vi "EyeFileExtraction.vi"() -> ()   [LabVIEW 2022 SP3]
uses:
  ViewData/-ReadEye/Header.ctl
  <vilib>/Utility/file.llb/Read Delimited Spreadsheet (string).vi
  <vilib>/Utility/file.llb/Read Delimited Spreadsheet (DBL).vi
  <userlib>/_OpenG.lib/array/array.llb/Sort 2D Array (DBL)__ogtk.vi
panel:
  in  "Save Folder Name":string="EyeFiles"
  in  "Only Real of Sum?":bool
  in  "Cut off":i32=50000
  in  "save folder path":path
  in  "Folder Override?":bool
  in  "Save All?":bool
  out "time diff":sgl[](graph)
  out "time stamp":sgl[](graph)
  in  "Split files?":bool
  out "Current File":string
  in  "IQ source":enum32{"GPU", "Verasonics", "None"}(radio)
  out "Current File Ct":i32
  in  "Enum":T1(ring)
  out "Header Size":i32[](array[numeric])
  out "Header clolumn names":string[](array[string])
  in  "Header as cluster":T2
  out "Header Values sorted":dbl[][](array[numeric])
  in  "Use Selected Files":bool
  in  "Listbox":i32[](listbox)
  in  "directory path of data and header file":path
  in  "search pattern":string="*_HeaderInfoRcv.txt"
  # "Naming must match up\nDo not change order in Matlab save !!!!!!!!!!!!!!!!!!!!!!!!!!!!!!"
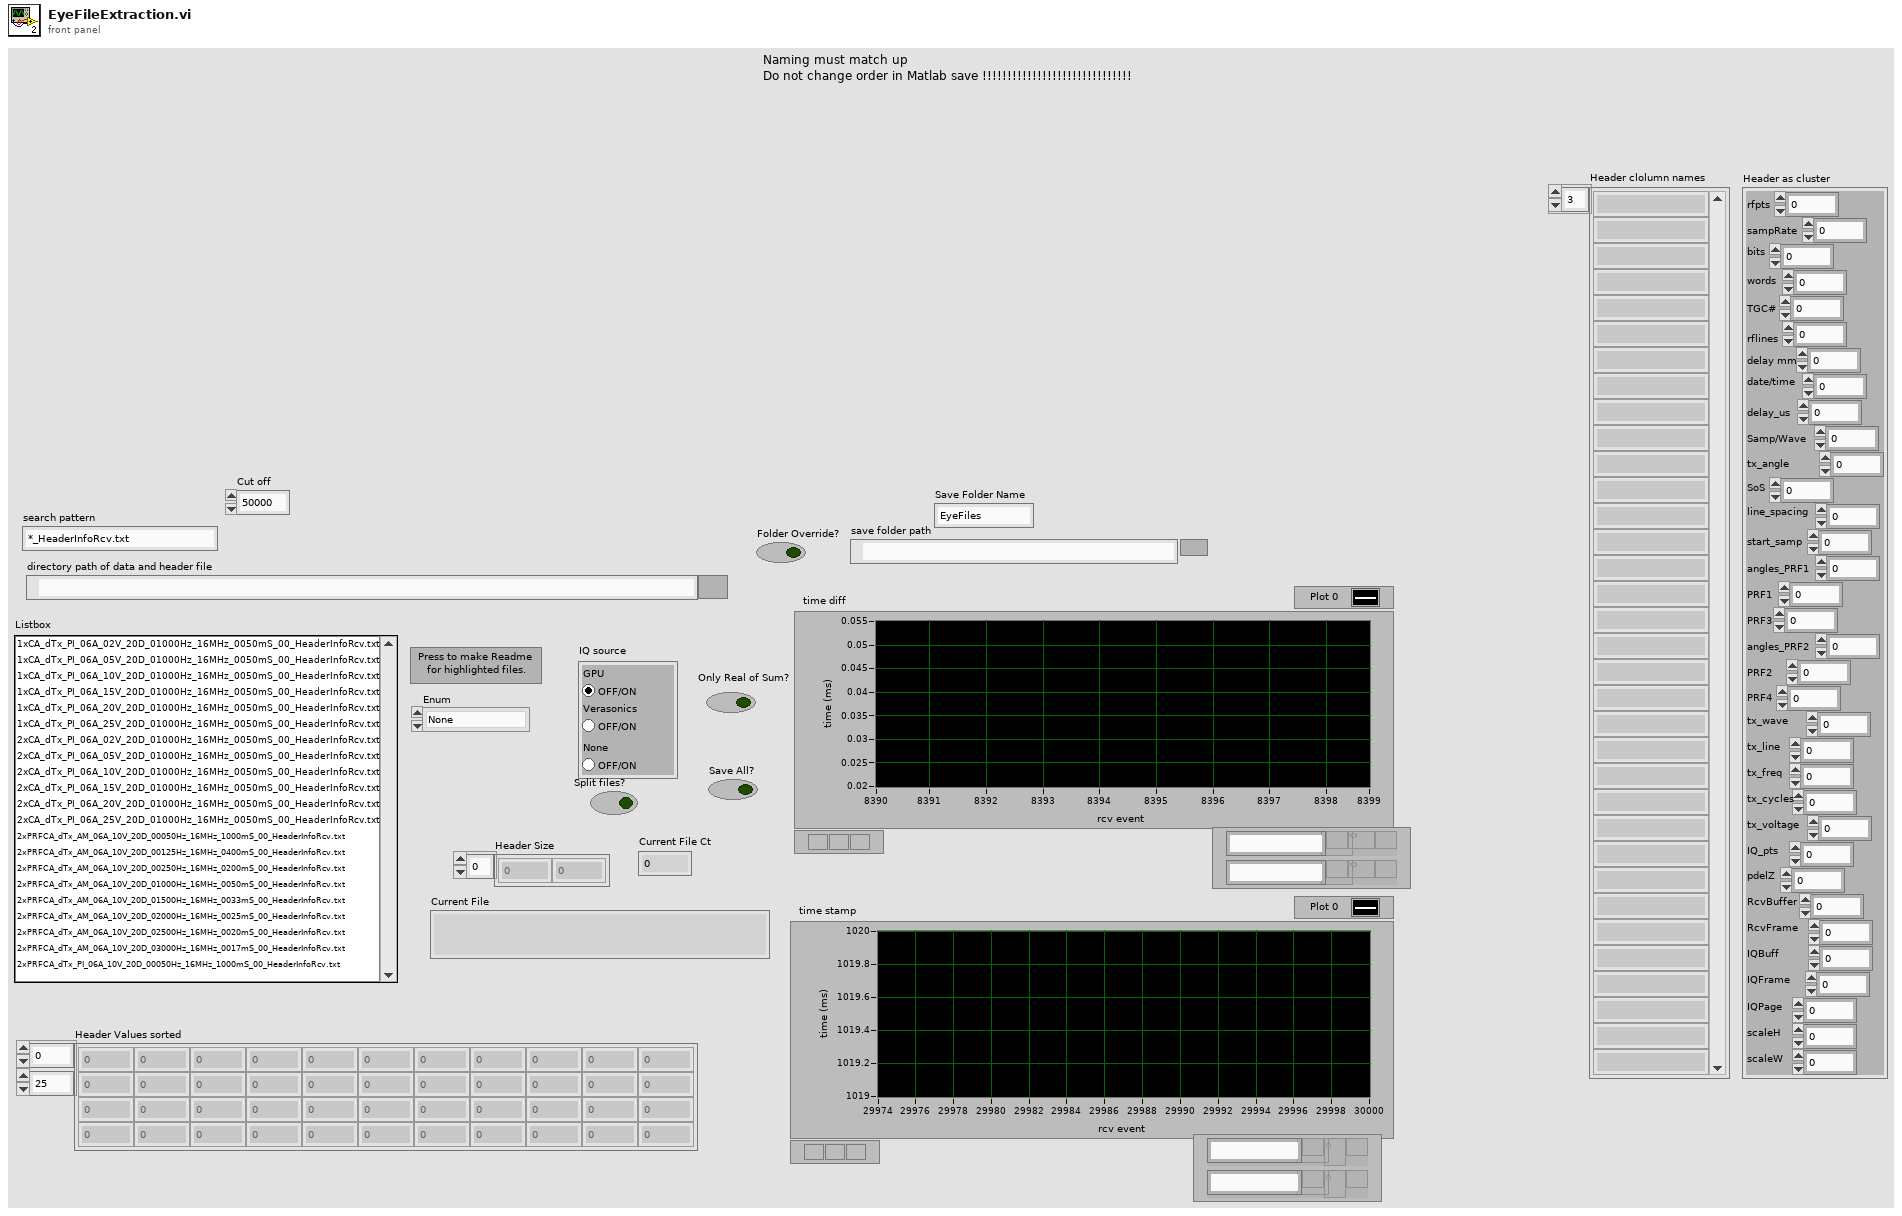
[diagram p1: front panel]
types:
  T1 = enum16{"None", "Save RF", "Save IQAll", "Save IQSum", "Save IQSumReal", "Save Img", "Time Stamps", "unused"}
  T2 = cluster{"rfpts":dbl, "sampRate":dbl, "bits":dbl, "words":dbl, "TGC#":dbl, "rflines":dbl, "delay mm":dbl, "date/time":dbl, "delay_us":dbl, "Samp/Wave":dbl, "tx_angle":dbl, "SoS":dbl, "line_spacing":dbl, "start_samp":dbl, "angles_PRF1":dbl, "PRF1":dbl, "PRF3":dbl, "angles_PRF2":dbl, "PRF2":dbl, "PRF4":dbl, "tx_wave":dbl, "tx_line":dbl, "tx_freq":dbl, "tx_cycles":dbl, "tx_voltage":dbl, "IQ_pts":dbl, "pdelZ":dbl, "RcvBuffer":dbl, "RcvFrame":dbl, "IQBuff":dbl, "IQFrame":dbl, "IQPage":dbl, "scaleH":dbl, "scaleW":dbl}
  T3 = typedef "Header.ctl" = cluster{"header info":cluster{"Header":string, "Head length":i16}, "A/D info":cluster{"# rf points per line":u16, "# lines per scan":u16, "sample rate MHz":u16, "# A/D bits":i16, "# bytes per A/D":u16, "TGC Flag":u16, "A/D Type":string}, "Tranducer Info":cluster{"bandwidth":sgl, "center freq":sgl, "start freq":sgl, "ID":i32}, "Scan Info":cluster{"delay":sgl, "pivot distance":sgl, "sector scan angle":sgl, "operator":string, "Scan Mode":string, "location":string}, "Time/Date Info":cluster{"date":string, "time":string}, "RF Info":cluster{"RF file name":string, "RF file att":string, "RF cal file name":string, "RF cal file att":string}, "Patient Info":cluster{"ID":string, "extended ID":string, "age":u16, "sex":string, "previously\nscanned":string, "PSA":sgl, "LOS":u8, "Ethnicty 2":u8, "Race":u8}, "Tissue Type":cluster{"organ":i16, "disease type":i16, "disease location":i16, "IQ_pts":u16, "RcvBuffer":u8, "RcvFrame":u16, "IQBuff":u8, "IQFrame":u16, "IQPage":u8}, "Votage scaling":cluster{"Digitizer (dB)":sgl, "Gain (dB)":sgl, "Atten (dB)":sgl}, "Comment":string, "Misc Info":cluster{"avg num":u16, "c speed":i16, "Div By or SF zones":i16, "XMIT CHS":u8, "RCV CHS":u8, "Xmit angle":sgl}, "Therapy Parameters":cluster{"Theraputic Freq (MHz)":sgl, "Time on (s)":sgl, "Therapy amplitude (mV)":sgl, "Lines Before":u16, "Lines After":u16}, "Scan Settings":cluster{"Energy (uJ or V)":u8, "Damp (Ohm) or Fc":u8, "HP Filt (KHz)":u8, "LP Filt (MHz)":u8, "Gain (db)":u8, "prf (kHz)":sgl, "Distance between\nscan lines (um)":u16, "Distance between\nscan planes (um)":u16, "Scan line gap (um)":sgl, "Scan plane gap (um)":sgl}, "Compression Parameters":cluster{"F1 (MHz)":sgl, "F2 (MHz)":sgl, "% taper":sgl, "duration":sgl}, "Patient Info Xtra":cluster{"First Name":string, "Last Name":string, "Notes":string}, "ROI Box":u16[]}
  T4 = enum16{"big-endian, network order", "native, host order", "little-endian"}
  T5 = enum16{"open", "replace", "create", "open or create", "replace or create", "replace or create with confirmation"}
  T6 = cluster{"Sorted Array out[0]":dbl, "Sorted Array out[1]":dbl, "Sorted Array out[2]":dbl, "Sorted Array out[3]":dbl, "Sorted Array out[4]":dbl, "Sorted Array out[5]":dbl, "Sorted Array out[6]":dbl, "Sorted Array out[7]":dbl, "Sorted Array out[8]":dbl, "Sorted Array out[9]":dbl, "Sorted Array out[10]":dbl, "Sorted Array out[11]":dbl, "Sorted Array out[12]":dbl, "Sorted Array out[13]":dbl, "Sorted Array out[14]":dbl, "Sorted Array out[15]":dbl, "Sorted Array out[16]":dbl, "Sorted Array out[17]":dbl, "Sorted Array out[18]":dbl, "Sorted Array out[19]":dbl, "Sorted Array out[20]":dbl, "Sorted Array out[21]":dbl, "Sorted Array out[22]":dbl, "Sorted Array out[23]":dbl, "Sorted Array out[24]":dbl, "Sorted Array out[25]":dbl, "Sorted Array out[26]":dbl, "Sorted Array out[27]":dbl, "Sorted Array out[28]":dbl, "Sorted Array out[29]":dbl, "Sorted Array out[30]":dbl, "Sorted Array out[31]":dbl, "Sorted Array out[32]":dbl, "Sorted Array out[33]":dbl, "Sorted Array out[34]":dbl}
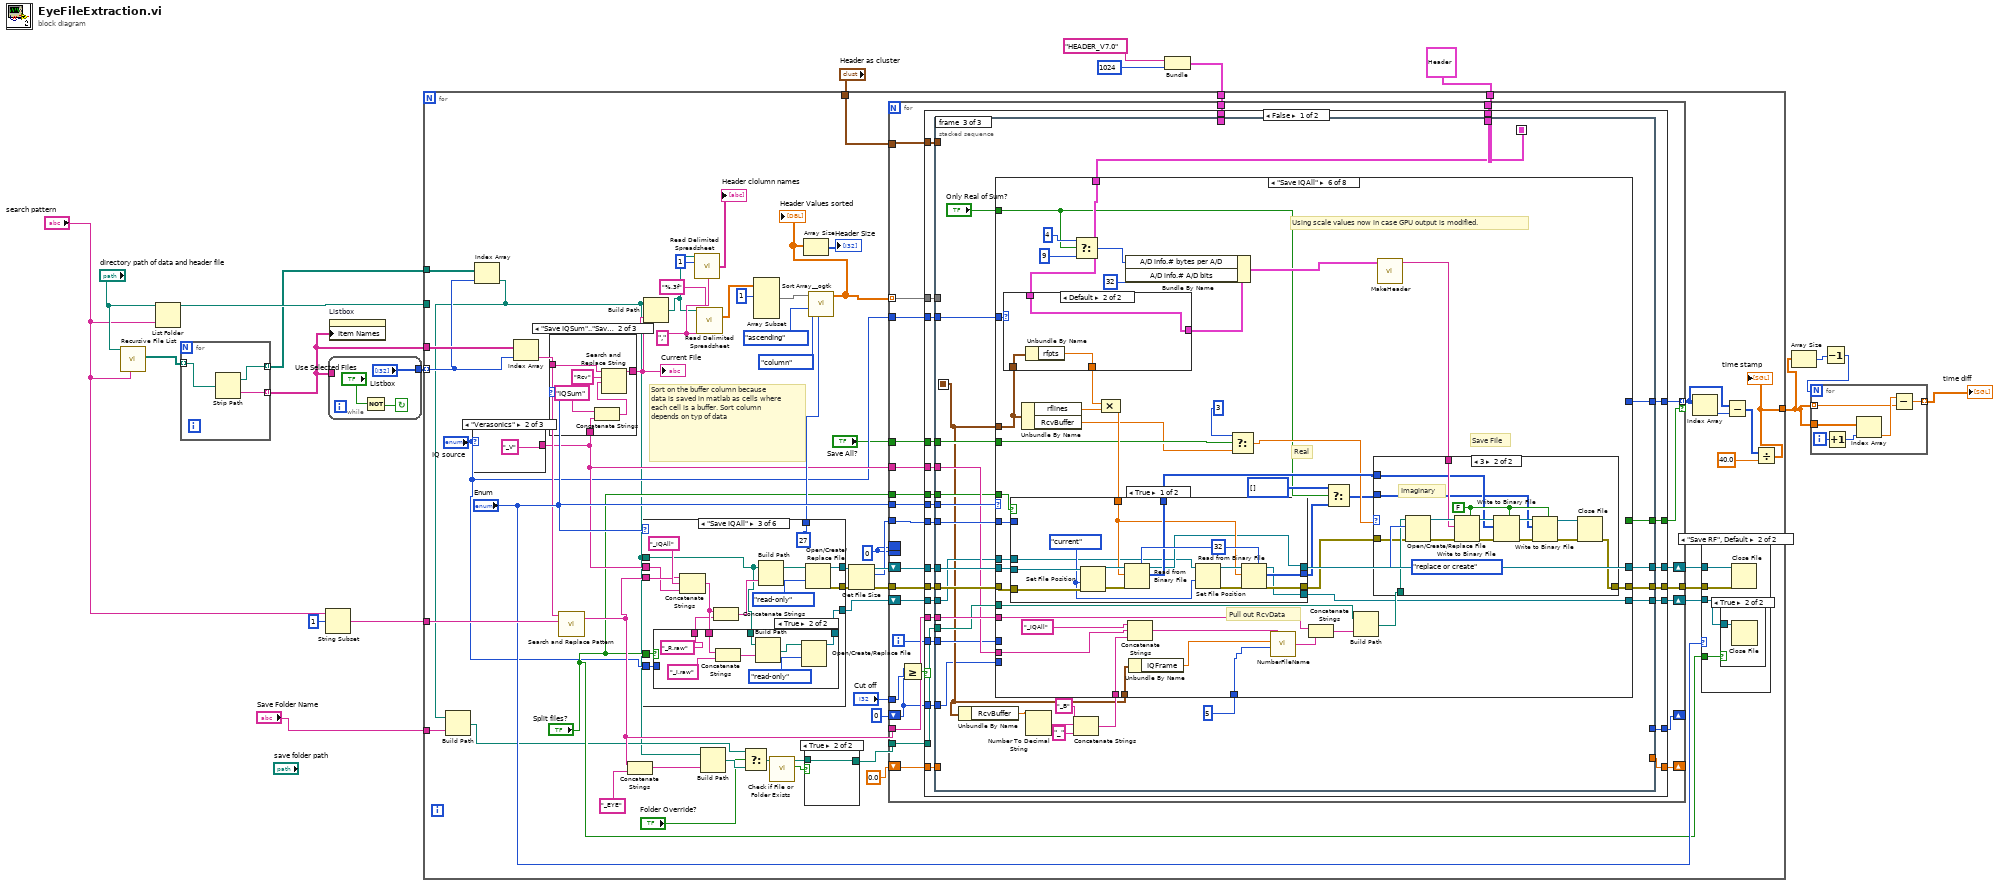
[diagram p0: block diagram]
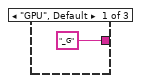
[diagram p2: hidden frame]
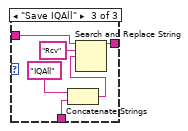
[diagram p5: hidden frame]
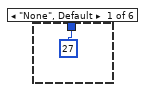
[diagram p8: hidden frame]
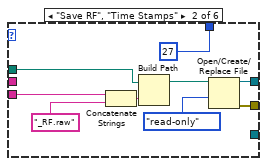
[diagram p9: hidden frame]
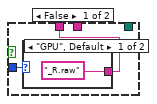
[diagram p10: hidden frame]
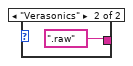
[diagram p11: hidden frame]
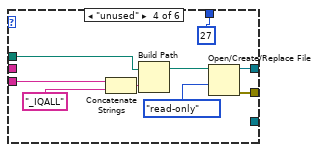
[diagram p12: hidden frame]
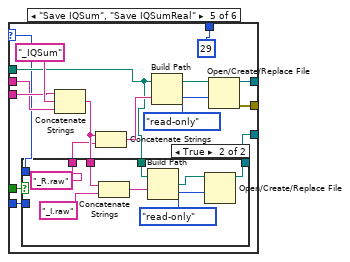
[diagram p13: hidden frame]
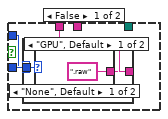
[diagram p14: hidden frame]
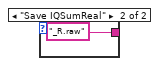
[diagram p15: hidden frame]
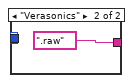
[diagram p16: hidden frame]
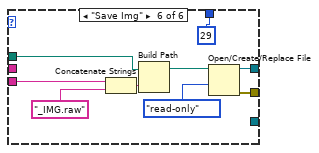
[diagram p17: hidden frame]
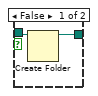
[diagram p18: hidden frame]
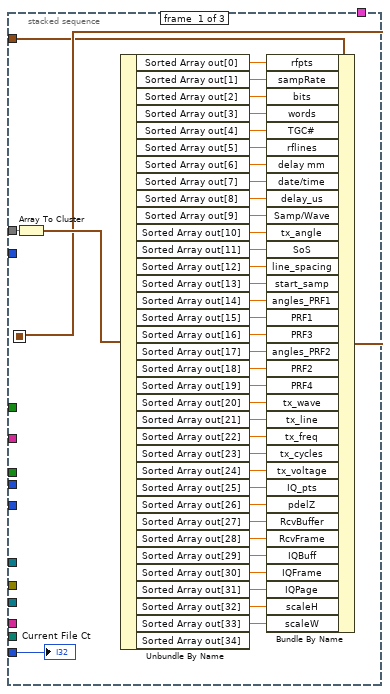
[diagram p19: hidden frame]
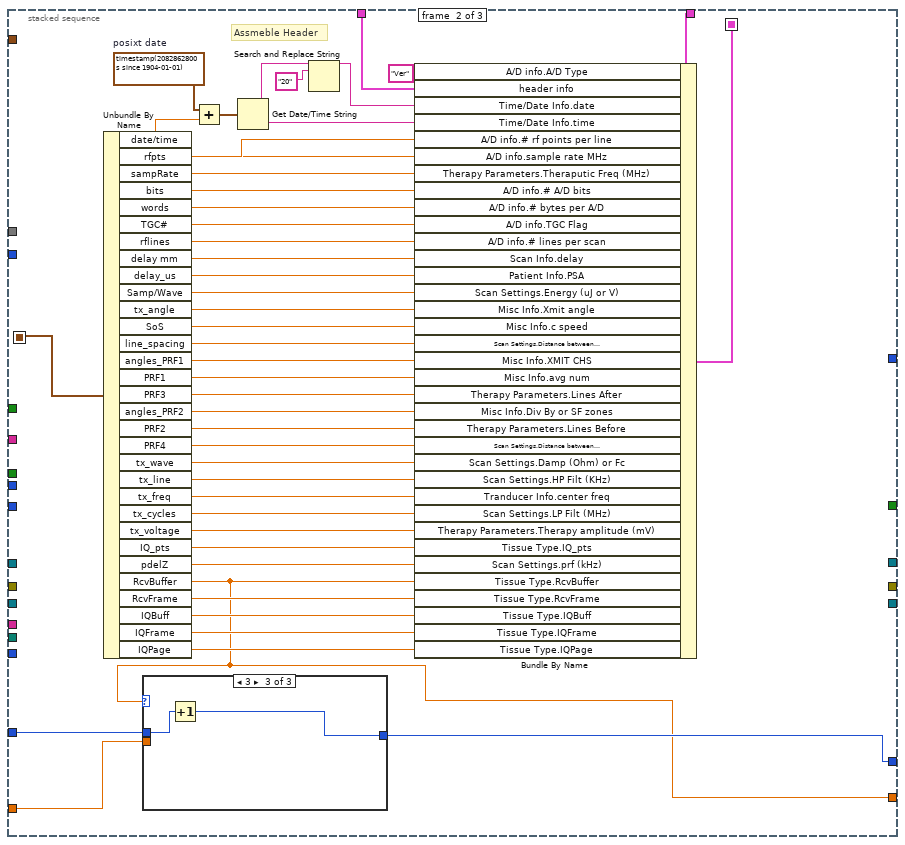
[diagram p20: hidden frame]
diagram:
  n1 = call <vilib>:"Recursive File List.vi"("pattern"="search pattern", "Folder Path"="directory path of data and header file") -> ("All Files in Dir"=w4:path[])  [unwired: 5 in, 4 out]
  n2 = List Folder(path="directory path of data and header file", pattern="search pattern") -> (path out=w7:path)  [unwired: 1 in, 4 out]
  n3 = for {
    tunnel: w4 -> [w22] mode=indexing
    tunnel: [w21] -> w3 mode=indexing
    tunnel: [w20] -> w2 mode=indexing
    n4 = Strip Path(path=w22) -> (stripped path=w20:path, name=w21:string)
  }
  n5 = String Subset(string="search pattern", offset (0)=1) -> (substring=w18:string)  [unwired: 1 in]
  n6 = while {
    tunnel: ["Listbox"] -> w19
    tunnel: w3 -> [_]
    stop <- w25 continue-if-true
    n7 = Not(x="Use Selected Files") -> (.not. x?=w25:bool)
  }
  n8 = property on="Listbox" class="LstBox (strict)"("Item Names"=w3) -> ()  [unwired: 2 in, 2 out]
  n9 = Bundle("HEADER_V7.0", 1024) -> (w13:cluster{string, i32})  [unwired: 1 in]
  n10 = for {
    tunnel: w19 -> [w28] mode=indexing
    tunnel: w3 -> [w82]
    tunnel: w7 -> [_]
    tunnel: w18 -> [w73]
    tunnel: "Header as cluster" -> [w79]
    tunnel: T3 {"header info"={"Header"="", "Head length"=0}, "A/D info"={"# rf points per line"=0, "# lines per scan"=0, "sample rate MHz"=0, "# A/D bits"=0, "# bytes per A/D"=0, "TGC Flag"=0, "A/D Type"=""}, "Tranducer Info"={"bandwidth"=0.0, "center freq"=0.0, "start freq"=0.0, "ID"=0}, "Scan Info"={"delay"=0.0, "pivot distance"=0.0, "sector scan angle"=0.0, "operator"="", "Scan Mode"="", "location"=""}, "Time/Date Info"={"date"="", "time"=""}, "RF Info"={"RF file name"="", "RF file att"="", "RF cal file name"="", "RF cal file att"=""}, "Patient Info"={"ID"="", "extended ID"="", "age"=0, "sex"="", "previously\nscanned"="", "PSA"=0.0, "LOS"=1, "Ethnicty 2"=3, "Race"=3}, "Tissue Type"={"organ"=0, "disease type"=0, "disease location"=0, "IQ_pts"=0, "RcvBuffer"=0, "RcvFrame"=0, "IQBuff"=0, "IQFrame"=0, "IQPage"=0}, "Votage scaling"={"Digitizer (dB)"=0.0, "Gain (dB)"=0.0, "Atten (dB)"=0.0}, "Comment"="", "Misc Info"={"avg num"=0, "c speed"=0, "Div By or SF zones"=0, "XMIT CHS"=0, "RCV CHS"=0, "Xmit angle"=0.0}, "Therapy Parameters"={"Theraputic Freq (MHz)"=0.0, "Time on (s)"=0.0, "Therapy amplitude (mV)"=0.0, "Lines Before"=0, "Lines After"=0}, "Scan Settings"={"Energy (uJ or V)"=0, "Damp (Ohm) or Fc"=0, "HP Filt (KHz)"=0, "LP Filt (MHz)"=0, "Gain (db)"=0, "prf (kHz)"=0.0, "Distance between\nscan lines (um)"=0, "Distance between\nscan planes (um)"=0, "Scan line gap (um)"=0.0, "Scan plane gap (um)"=0.0}, "Compression Parameters"={"F1 (MHz)"=0.0, "F2 (MHz)"=0.0, "% taper"=0.0, "duration"=0.0}, "Patient Info Xtra"={"First Name"="", "Last Name"="", "Notes"=""}, "ROI Box"=[0, 0, 0, 0]} ("Header In") -> [w75]
    tunnel: w13 -> [w67]
    tunnel: [w42] -> w10
    tunnel: "Save Folder Name" -> [w30]
    tunnel: w2 -> [w27]
    w34 = i64 0 ("offset (in bytes)")
    w77 = "," ("delimiter (\\t)")
    # "Sort on the buffer column because data is saved in matlab as cells where each cell is a buffer. Sort column depends on typ of data"
    n11 = case shown="\"Verasonics\"" "IQ source" {
      tunnel: ["_G" ("replace string (\"\")") "_V" ("replace string (\"\")") _] -> w51
      frame "GPU", Default {
      }
      frame "Verasonics" {
      }
      frame "None" {
      }
    }
    n12 = Index Array(array=w27, index=w28) -> (element=w26:path)
    n13 = Build Path(base path=w26, name or relative path=w30) -> (appended path=w29:path)
    n14 = Index Array(array=w82, index=w28) -> (element=w62:string)
    n15 = case shown="\"Save IQSum\"..\"Save Img\"" "Enum" {
      tunnel: w62 -> [w85 w90 w96]
      tunnel: [w85 w89 w95] -> w61
      tunnel: w51 -> [_ w86 w92]
      frame "None", Default {
      }
      frame "Save IQSum".."Save Img" {
        n16 = Concatenate Strings("IQSum" ("replace string (\"\")"), w86) -> (w87:string)
        n17 = Search and Replace String(input string=w90, search string="Rcv", replace string=w87) -> (result string=w89:string)  [unwired: 5 in, 3 out]
      }
      frame "Save IQAll" {
        n18 = Concatenate Strings("IQAll" ("replace string (\"\")"), w92) -> (w93:string)
        n19 = Search and Replace String(input string=w96, search string="Rcv", replace string=w93) -> (result string=w95:string)  [unwired: 5 in, 3 out]
      }
    }
    "Current File" <- w61
    n20 = call <vilib>:"Search and Replace Pattern.vi"("string"=w62, "regular expression (\"\")"=w73) -> ("result string"=w66:string)  [unwired: 3 in, 1 out]
    n21 = Concatenate Strings(w66, "_EYE") -> (w72:string)
    n22 = case shown="\"Save IQAll\"" "Enum" {
      selector: "Enum" -> [_ _ _ _ w149 _]
      tunnel: w66 -> [_ w110 w126 w146 w163 w187]
      tunnel: [_ w108 w124 w144 w161 w185] -> w55
      tunnel: [_ w107 w123 w143 w160 w184] -> w54
      tunnel: w26 -> [_ w105 w117 w141 w154 w182]
      tunnel: [u32 27 ("Column/Row to Sort By") u32 27 ("Column/Row to Sort By") u32 27 ("Column/Row to Sort By") u32 27 ("Column/Row to Sort By") u32 29 ("Column/Row to Sort By") u32 29 ("Column/Row to Sort By")] -> w56
      tunnel: w51 -> [_ _ w120 _ w157 _]
      tunnel: [_ _ w116 _ w153 _] -> w50
      tunnel: "Split files?" -> [_ _ w115 _ w152 _]
      tunnel: "IQ source" -> [_ _ w113 _ w150 _]
      frame "None", Default {
      }
      frame "Save RF", "Time Stamps" {
        n23 = Concatenate Strings(w110, "_RF.raw") -> (w112:string)
        n24 = Build Path(base path=w105, name or relative path=w112) -> (appended path=w109:path)
        n25 = Open/Create/Replace File(file path (use dialog)=w109, access (0:read/write)=enum16{"read/write", "read-only", "write-only"}."read-only") -> (refnum out=w108:refnum<file>, error out=w107:errorcluster)  [unwired: 4 in, 1 out]
      }
      frame "Save IQAll" {
        n26 = Concatenate Strings(w126, "_IQAll", w120) -> (w119:string)
        n27 = case shown="True" w115 {
          tunnel: w119 -> [_ w139]
          tunnel: w117 -> [_ w135]
          tunnel: [_ w133] -> w116
          tunnel: [w128 "_R.raw"] -> w114
          tunnel: w113 -> [w129 _]
          frame False {
            n28 = case shown="\"GPU\", Default" w129 {
              tunnel: ["_R.raw" ".raw"] -> w128
              frame "GPU", Default {
              }
              frame "Verasonics" {
              }
            }
          }
          frame True {
            n29 = Concatenate Strings(w139, "_I.raw") -> (w136:string)
            n30 = Build Path(base path=w135, name or relative path=w136) -> (appended path=w134:path)
            n31 = Open/Create/Replace File(file path (use dialog)=w134, access (0:read/write)=enum16{"read/write", "read-only", "write-only"}."read-only") -> (refnum out=w133:refnum<file>)  [unwired: 4 in, 2 out]
          }
        }
        n32 = Concatenate Strings(w119, w114) -> (w118:string)
        n33 = Build Path(base path=w117, name or relative path=w118) -> (appended path=w125:path)
        n34 = Open/Create/Replace File(file path (use dialog)=w125, access (0:read/write)=enum16{"read/write", "read-only", "write-only"}."read-only") -> (refnum out=w124:refnum<file>, error out=w123:errorcluster)  [unwired: 4 in, 1 out]
      }
      frame "unused" {
        n35 = Concatenate Strings(w146, "_IQALL") -> (w148:string)
        n36 = Build Path(base path=w141, name or relative path=w148) -> (appended path=w145:path)
        n37 = Open/Create/Replace File(file path (use dialog)=w145, access (0:read/write)=enum16{"read/write", "read-only", "write-only"}."read-only") -> (refnum out=w144:refnum<file>, error out=w143:errorcluster)  [unwired: 4 in, 1 out]
      }
      frame "Save IQSum", "Save IQSumReal" {
        n38 = Concatenate Strings(w163, "_IQSum", w157) -> (w156:string)
        n39 = case shown="True" w152 {
          tunnel: w156 -> [_ w180]
          tunnel: w154 -> [_ w176]
          tunnel: [_ w174] -> w153
          tunnel: [w166 "_R.raw"] -> w151
          tunnel: w150 -> [w167 _]
          tunnel: w149 -> [w165 _]
          frame False {
            n40 = case shown="\"GPU\", Default" w167 {
              tunnel: [w169 ".raw"] -> w166
              tunnel: w165 -> [w168 _]
              frame "GPU", Default {
                n41 = case shown="\"None\", Default" w168 {
                  tunnel: [".raw" "_R.raw"] -> w169
                  frame "None", Default {
                  }
                  frame "Save IQSumReal" {
                  }
                }
              }
              frame "Verasonics" {
              }
            }
          }
          frame True {
            n42 = Concatenate Strings(w180, "_I.raw") -> (w177:string)
            n43 = Build Path(base path=w176, name or relative path=w177) -> (appended path=w175:path)
            n44 = Open/Create/Replace File(file path (use dialog)=w175, access (0:read/write)=enum16{"read/write", "read-only", "write-only"}."read-only") -> (refnum out=w174:refnum<file>)  [unwired: 4 in, 2 out]
          }
        }
        n45 = Concatenate Strings(w156, w151) -> (w155:string)
        n46 = Build Path(base path=w154, name or relative path=w155) -> (appended path=w162:path)
        n47 = Open/Create/Replace File(file path (use dialog)=w162, access (0:read/write)=enum16{"read/write", "read-only", "write-only"}."read-only") -> (refnum out=w161:refnum<file>, error out=w160:errorcluster)  [unwired: 4 in, 1 out]
      }
      frame "Save Img" {
        n48 = Concatenate Strings(w187, "_IMG.raw") -> (w189:string)
        n49 = Build Path(base path=w182, name or relative path=w189) -> (appended path=w186:path)
        n50 = Open/Create/Replace File(file path (use dialog)=w186, access (0:read/write)=enum16{"read/write", "read-only", "write-only"}."read-only") -> (refnum out=w185:refnum<file>, error out=w184:errorcluster)  [unwired: 4 in, 1 out]
      }
    }
    n51 = Build Path(base path=w26, name or relative path=w61) -> (appended path=w32:path)
    n52 = call-poly <vilib>:"Read Delimited Spreadsheet.vi"("file path (dialog if empty)"=w32, "number of rows (all:-1)"=1, "delimiter (\\t)"=w77) -> ("first row"=→"Header clolumn names":string[])  [unwired: 7 in, 5 out]
    n53 = call-poly <vilib>:"Read Delimited Spreadsheet.vi"("file path (dialog if empty)"=w32, "format (%.3f)"="%.3f", "delimiter (\\t)"=w77) -> ("all rows"=w81:dbl[][])  [unwired: 7 in, 5 out]
    n54 = Build Path(base path=w26, name or relative path=w72) -> (appended path=w40:path)
    n55 = Select(t=w29, s="Folder Override?", f=w40) -> (s? t:f=w39:path)
    n56 = Array Subset(array=w81, index (row)=1 ("index")) -> (w58:dbl[][])  [unwired: 3 in]
    n57 = call <vilib>:"Check if File or Folder Exists.vi"("path"=w39) -> ("file or folder exists?"=w69:bool, "dup path"=w68:path)  [unwired: 8 in, 1 out]
    n58 = case shown="True" w69 {
      tunnel: [w191 w192] -> w70
      tunnel: w68 -> [w190 w192]
      frame False {
        n59 = Create Folder(path (use dialog)=w190) -> (created path=w191:path)  [unwired: 2 in, 2 out]
      }
      frame True {
      }
    }
    n60 = call-poly <userlib>:"Sort Array__ogtk.vi"("Column/Row to Sort By"=w56, "Sort By in"=enum16{"row", "column"}."column", "Order"=enum16{"ascending", "descending"}."ascending", "Array in"=w58) -> ("Sorted Array out"=w57:dbl[][])  [unwired: 4 in, 3 out]
    "Header Values sorted" <- w57
    n61 = Array Size(array=w57) -> (size(s)=→"Header Size":i32[])
    n62 = Get File Size(file=w55, error in=w54) -> (refnum out=w53:refnum<file>, size (in bytes)=w35:i64, 0:w52:errorcluster)
    n63 = for {
      tunnel: w57 -> [w210] mode=indexing
      tunnel: w79 -> [w209]
      tunnel: w75 -> [w219]
      tunnel: w70 -> [w216]
      tunnel: w66 -> [w217]
      tunnel: w67 -> [w218]
      tunnel: w52 -> [w214]
      tunnel: [w212] -> w65
      tunnel: "Enum" -> [w211]
      shift-right: [w213] -> w64
      shift-left: w53 -> [w215]
      tunnel: w35 -> [w208]
      border: w34 -> [_]
      tunnel: w51 -> [w207]
      tunnel: "Split files?" -> [w206]
      shift-right: [w204] -> w48
      shift-left: w50 -> [w205]
      tunnel: "IQ source" -> [w203]
      tunnel: [w202] -> w45 mode=indexing if=w201
      tunnel: "Save All?" -> [w200]
      tunnel: "Cut off" -> [w198]
      shift-right: [w197] -> _
      shift-left: 0 ("IQFrame") -> [w194]
      border: w34 -> [_]
      shift-right: [w193] -> _
      shift-left: 0.0 ("IQFrame") -> [w195]
      i -> [w199]
      n64 = Greater Or Equal?(x=w194, y=w198) -> (x >= y?=w196:bool)
      n65 = case shown="False" w196 {
        tunnel: w219 -> [w244 _]
        tunnel: w218 -> [w243 _]
        tunnel: w217 -> [w242 _]
        tunnel: w199 -> [w241 _]
        tunnel: w216 -> [w240 _]
        tunnel: w215 -> [w239 w883]
        tunnel: w214 -> [w238 w882]
        tunnel: [w237 w883] -> w213
        tunnel: [w236 w882] -> w212
        tunnel: w211 -> [w235 _]
        tunnel: w210 -> [w234 _]
        tunnel: w209 -> [w233 _]
        tunnel: w208 -> [w232 _]
        tunnel: w207 -> [w231 _]
        tunnel: w206 -> [w230 _]
        tunnel: w205 -> [w229 w881]
        tunnel: [w228 w881] -> w204
        tunnel: w203 -> [w227 _]
        tunnel: [w226 _] -> w202
        tunnel: [w225 FALSE] -> w201
        tunnel: w200 -> [w224 _]
        tunnel: [w223 w878] -> w197
        tunnel: w195 -> [w222 w879]
        tunnel: w194 -> [w221 w878]
        tunnel: [w220 w879] -> w193
        frame False {
          n66 = stacked-sequence {
            seq-local: [_ w297 _] -> [_ _ w365]
            seq-local: [w249 _ _] -> [_ w296 w340]
            tunnel: w244 -> [_ w328 _]
            tunnel: w243 -> [_ w302 _]
            tunnel: w242 -> [_ _ w364]
            tunnel: w241 -> [w247 _ w346]
            tunnel: w240 -> [_ _ w363]
            tunnel: w239 -> [_ _ w362]
            tunnel: w238 -> [_ _ w361]
            tunnel: [_ _ w360] -> w237
            tunnel: [_ _ w359] -> w236
            tunnel: w235 -> [_ _ w358]
            tunnel: w234 -> [w251 _ _]
            tunnel: w233 -> [w248 _ _]
            tunnel: w232 -> [_ _ w353]
            tunnel: w231 -> [_ _ w351]
            tunnel: w230 -> [_ _ w350]
            tunnel: w229 -> [_ _ w349]
            tunnel: [_ _ w348] -> w228
            tunnel: w227 -> [_ _ w347]
            tunnel: [_ _ w345] -> w226
            tunnel: [_ _ w344] -> w225
            tunnel: w224 -> [_ _ w343]
            tunnel: [_ w285 _] -> w223
            tunnel: w222 -> [_ w287 _]
            tunnel: w221 -> [_ w286 w339]
            tunnel: [_ w284 _] -> w220
            frame #0 {
              n67 = Array To Cluster(array=w251) -> (cluster=w250:T6)
              n68 = Unbundle By Name(w250) -> ("Sorted Array out[0]"=w283:dbl, "Sorted Array out[1]"=w282:dbl, "Sorted Array out[2]"=w281:dbl, "Sorted Array out[3]"=w280:dbl, "Sorted Array out[4]"=w279:dbl, "Sorted Array out[5]"=w278:dbl, "Sorted Array out[6]"=w277:dbl, "Sorted Array out[7]"=w276:dbl, "Sorted Array out[8]"=w275:dbl, "Sorted Array out[9]"=w274:dbl, "Sorted Array out[10]"=w273:dbl, "Sorted Array out[11]"=w272:dbl, "Sorted Array out[12]"=w271:dbl, "Sorted Array out[13]"=w270:dbl, "Sorted Array out[14]"=w269:dbl, "Sorted Array out[15]"=w268:dbl, "Sorted Array out[16]"=w267:dbl, "Sorted Array out[17]"=w266:dbl, "Sorted Array out[18]"=w265:dbl, "Sorted Array out[19]"=w264:dbl, "Sorted Array out[20]"=w263:dbl, "Sorted Array out[21]"=w262:dbl, "Sorted Array out[22]"=w261:dbl, "Sorted Array out[23]"=w260:dbl, "Sorted Array out[24]"=w259:dbl, "Sorted Array out[25]"=w258:dbl, "Sorted Array out[26]"=w257:dbl, "Sorted Array out[27]"=w256:dbl, "Sorted Array out[28]"=w255:dbl, "Sorted Array out[29]"=w252:dbl, "Sorted Array out[30]"=w253:dbl, "Sorted Array out[31]"=w254:dbl, "Sorted Array out[32]"=w246:dbl, "Sorted Array out[33]"=w245:dbl)  [unwired: 1 out]
              n69 = Bundle By Name(cluster=w248, "rfpts"=w283, "sampRate"=w282, "bits"=w281, "words"=w280, "TGC#"=w279, "rflines"=w278, "delay mm"=w277, "date/time"=w276, "delay_us"=w275, "Samp/Wave"=w274, "tx_angle"=w273, "SoS"=w272, "line_spacing"=w271, "start_samp"=w270, "angles_PRF1"=w269, "PRF1"=w268, "PRF3"=w267, "angles_PRF2"=w266, "PRF2"=w265, "PRF4"=w264, "tx_wave"=w263, "tx_line"=w262, "tx_freq"=w261, "tx_cycles"=w260, "tx_voltage"=w259, "IQ_pts"=w258, "pdelZ"=w257, "RcvBuffer"=w256, "RcvFrame"=w255, "IQBuff"=w252, "IQFrame"=w253, "IQPage"=w254, "scaleH"=w246, "scaleW"=w245) -> (w249:T2)
              "Current File Ct" <- w247
            }
            frame #1 {
              w313 = timestamp(2082862800 s since 1904-01-01)  # posixt date
              # "Assmeble Header"
              n70 = Unbundle By Name(w296) -> ("date/time"=w314:dbl, "rfpts"=w289:dbl, "sampRate"=w288:dbl, "bits"=w309:dbl, "words"=w327:dbl, "TGC#"=w326:dbl, "rflines"=w325:dbl, "delay mm"=w324:dbl, "delay_us"=w323:dbl, "Samp/Wave"=w322:dbl, "tx_angle"=w303:dbl, "SoS"=w317:dbl, "line_spacing"=w304:dbl, "angles_PRF1"=w321:dbl, "PRF1"=w308:dbl, "PRF3"=w320:dbl, "angles_PRF2"=w318:dbl, "PRF2"=w319:dbl, "PRF4"=w307:dbl, "tx_wave"=w306:dbl, "tx_line"=w305:dbl, "tx_freq"=w301:dbl, "tx_cycles"=w300:dbl, "tx_voltage"=w299:dbl, "IQ_pts"=w295:dbl, "pdelZ"=w294:dbl, "RcvBuffer"=w284:dbl, "RcvFrame"=w293:dbl, "IQBuff"=w292:dbl, "IQFrame"=w291:dbl, "IQPage"=w290:dbl)
              n71 = case shown="3" w284 {
                selector: w284 -> [_ w330 _]
                tunnel: w287 -> [_ w336 _]
                tunnel: w286 -> [w329 w333 w338]
                tunnel: [w329 w332 w337] -> w285
                frame 0, Default {
                }
                frame 6 {
                  n72 = Increment(x=w333) -> (x+1=w334:i32)
                  n73 = Equal?(x=w330, y=w336) -> (x = y?=w335:bool)
                  n74 = Select(t=w334, s=w335, f=0) -> (s? t:f=w332:i32)
                }
                frame 3 {
                  n75 = Increment(x=w338) -> (x+1=w337:i32)
                }
              }
              n76 = Add(x=w313, y=w314) -> (x+y=w316:timestamp)
              n77 = Get Date/Time String(seconds (now)=w316) -> (date string=w312:string, time string=w315:string)  [unwired: 2 in]
              n78 = Search and Replace String(input string=w312, search string="20") -> (result string=w310:string)  [unwired: 2 in, 7 out]
              n79 = Bundle By Name(cluster=w328, "A/D info.A/D Type"="Ver", "header info"=w302, "Time/Date Info.date"=w310, "Time/Date Info.time"=w315, "A/D info.# rf points per line"=w289, "A/D info.sample rate MHz"=w288, "Therapy Parameters.Theraputic Freq (MHz)"=w288, "A/D info.# A/D bits"=w309, "A/D info.# bytes per A/D"=w327, "A/D info.TGC Flag"=w326, "A/D info.# lines per scan"=w325, "Scan Info.delay"=w324, "Patient Info.PSA"=w323, "Scan Settings.Energy (uJ or V)"=w322, "Misc Info.Xmit angle"=w303, "Misc Info.c speed"=w317, "Scan Settings.Distance between\nscan lines (um)"=w304, "Misc Info.XMIT CHS"=w321, "Misc Info.avg num"=w308, "Therapy Parameters.Lines After"=w320, "Misc Info.Div By or SF zones"=w318, "Therapy Parameters.Lines Before"=w319, "Scan Settings.Distance between\nscan planes (um)"=w307, "Scan Settings.Damp (Ohm) or Fc"=w306, "Scan Settings.HP Filt (KHz)"=w305, "Tranducer Info.center freq"=w301, "Scan Settings.LP Filt (MHz)"=w300, "Therapy Parameters.Therapy amplitude (mV)"=w299, "Tissue Type.IQ_pts"=w295, "Scan Settings.prf (kHz)"=w294, "Tissue Type.RcvBuffer"=w284, "Tissue Type.RcvFrame"=w293, "Tissue Type.IQBuff"=w292, "Tissue Type.IQFrame"=w291, "Tissue Type.IQPage"=w290) -> (w297:T3)
            }
            frame #2 {
              n80 = Unbundle By Name(w340) -> ("RcvBuffer"=w341:dbl)
              n81 = Number To Decimal String(number=w341) -> (decimal integer string=w357:string)  [unwired: 1 in]
              n82 = Concatenate Strings("_B" ("string"), w357, "_" ("string")) -> (w355:string)
              n83 = case shown="\"Save IQAll\"" w358 {
                tunnel: w365 -> [_ w372 _ w501 w559 w664 w792 w824]
                tunnel: w340 -> [_ w407 w487 w518 w561 w666 w779 w823]
                tunnel: w364 -> [_ w403 _ w527 w584 w689 w798 w830]
                tunnel: w363 -> [_ w402 _ w526 w583 w688 w797 w829]
                tunnel: w362 -> [w367 w400 w457 w513 w572 w658 w770 w828]
                tunnel: w361 -> [w366 w399 w454 w512 w571 w676 w769 w827]
                tunnel: [w367 w398 w480 w504 w582 w687 w796 w826] -> w360
                tunnel: [w366 w395 w479 w517 w576 w680 w777 w825] -> w359
                tunnel: w355 -> [_ w393 _ w515 w575 w679 w774 w821]
                tunnel: w353 -> [_ _ _ _ w573 w677 w772 _]
                tunnel: 5 ("Digits") -> [_ w391 _ w508 w569 w674 w757 w820]
                tunnel: w351 -> [_ _ _ w506 w567 w672 _ _]
                tunnel: w350 -> [_ _ _ _ w565 w670 _ _]
                tunnel: w349 -> [_ _ _ w500 w564 w669 _ _]
                tunnel: [_ _ _ w500 w563 w668 _ _] -> w348
                tunnel: w347 -> [_ _ _ _ w562 w667 _ _]
                tunnel: w346 -> [_ _ w453 _ _ _ _ _]
                tunnel: [_ w390 w486 _ _ _ _ _] -> w345
                tunnel: [_ w385 w483 _ _ _ _ _] -> w344
                tunnel: w343 -> [_ w389 _ w497 w556 w661 _ _]
                tunnel: "Only Real of Sum?" -> [_ _ _ _ w546 w652 _ _]
                tunnel: w340 -> [_ _ _ w495 w545 w650 w755 w819]
                tunnel: w339 -> [_ w368 _ _ _ _ _ _]
                frame "None", Default {
                }
                frame "Save RF" {
                  # "Handle 2 smps case"
                  # "Pull out time stamp"
                  # "Save FIle"
                  # "Pull out RcvData"
                  n84 = Unbundle By Name(w407) -> ("angles_PRF1"=w380:dbl, "RcvFrame"=w384:dbl, "tx_line"=w369:dbl, "rfpts"=w374:dbl, "rflines"=w373:dbl, "RcvBuffer"=w387:dbl, "Samp/Wave"=w371:dbl)  [unwired: 1 out]
                  n85 = case shown="True" TRUE {
                    tunnel: w384 -> [_ w426]
                    tunnel: [_ w425] -> w383
                    tunnel: w369 -> [_ w423]
                    frame False {
                    }
                    frame True {
                      w424 = "" ("String")
                      n86 = call "NumberFileName.vi"("String"=w424, "Digits"=3, "File number"=w426) -> ("Numbered File"=w431:string)  [unwired: 1 in]
                      n87 = Concatenate Strings("_F" ("file name"), w431) -> (w427:string)
                      n88 = call "NumberFileName.vi"("String"=w424, "Digits"=2, "File number"=w423) -> ("Numbered File"=w429:string)  [unwired: 1 in]
                      n89 = Concatenate Strings(w427, "_L" ("file name"), w429) -> (w425:string)
                    }
                  }
                  n90 = Increment(x=w380) -> (x+1=w370:dbl)
                  n91 = Concatenate Strings("_RF" ("file name"), w393) -> (w392:string)
                  n92 = Select(t=3, s=w389, f=w387) -> (s? t:f=w386:dbl)
                  n93 = Subtract(x=w370, y=w369) -> ()  [unwired: 1 out]
                  n94 = Set File Position(refnum=w400, from (0:start)=enum16{"start", "end", "current"}."current", error in=w399) -> (refnum out=w408:refnum<file>, error out=w409:errorcluster)  [unwired: 1 in]
                  n95 = Multiply(x=w374, y=w373) -> (x*y=w411:dbl)
                  n96 = call "NumberFileName.vi"("String"="", "Digits"=w391, "File number"=w368, "file name"=w392) -> ("Numbered File"=w406:string)
                  n97 = Read from Binary File(5:i16 16 ("A/D info.# A/D bits"), 8:w409, 9:T4."little-endian" ("byte order (0:big-endian, network order)"), 10:w411, 11:w408) -> (0:w396:errorcluster, 2:w375:i16[], 3:w398:refnum<file>)  [unwired: 1 in, 1 out]
                  n98 = Concatenate Strings(w403, w406, w383, ".eye" ("String")) -> (w405:string)
                  n99 = case shown="2" w371 {
                    tunnel: w372 -> [w413 w422]
                    tunnel: [w413 w421] -> w378
                    tunnel: w375 -> [w414 w420]
                    tunnel: [w415 w419] -> w377
                    tunnel: w374 -> [w417 _]
                    tunnel: w373 -> [w416 _]
                    frame 0, Default {
                      n100 = Reshape Array(w414, w417, w416) -> (w418:i16[][])
                      n101 = Transpose 2D Array(2D array=w418) -> (transposed array=w415:i16[][])
                    }
                    frame 2 {
                      n102 = call "RF_SPW_Upsample.vi"("Header In"=w422, "RF Data In"=w420) -> ("Header Out"=w421:T3, "RF Out 2D"=w419:i16[][])  [unwired: 6 in, 2 out]
                    }
                  }
                  n103 = Build Path(base path=w402, name or relative path=w405) -> (appended path=w404:path)
                  n104 = call "MakeHeader.vi"("Header In"=w378) -> ("Header String"=w401:string)  [unwired: 6 in]
                  n105 = case shown="3" w386 {
                    tunnel: w377 -> [_ _ w450]
                    tunnel: T5."replace or create" ("operation (0:open)") -> [_ _ w447]
                    tunnel: w404 -> [_ _ w446]
                    tunnel: w401 -> [_ _ w445]
                    tunnel: w396 -> [w435 w437 w442]
                    tunnel: [w435 w437 w441] -> w395
                    tunnel: [FALSE TRUE TRUE] -> w385
                    frame 0, Default {
                    }
                    frame 5 {
                    }
                    frame 3 {
                      w439 = FALSE ("prepend array or string size? (T)")
                      n106 = Open/Create/Replace File(file path (use dialog)=w446, error in=w442, operation (0:open)=w447) -> (refnum out=w449:refnum<file>, error out=w448:errorcluster)  [unwired: 3 in, 1 out]
                      n107 = Write to Binary File(file (use dialog)=w449, data=w445, error in=w448, 5:w439) -> (refnum out=w452:refnum<file>, error out=w451:errorcluster)  [unwired: 2 in, 1 out]
                      n108 = Write to Binary File(file (use dialog)=w452, data=w450, error in=w451, 5:w439, 9:T4."little-endian" ("byte order (0:big-endian, network order)")) -> (refnum out=w444:refnum<file>, error out=w443:errorcluster)  [unwired: 1 in, 1 out]
                      n109 = Close File(refnum=w444, error in=w443) -> (error out=w441:errorcluster)  [unwired: 1 out]
                    }
                  }
                  n110 = call "VerasonicsTimeStamp.vi"("Array"=w377) -> ("Numeric"=w390:u32)  [unwired: 10 in]
                }
                frame "Time Stamps" {
                  w474 = 1 ("count (1)")
                  w470 = enum16{"start", "end", "current"}."start" ("from (0:start)")
                  w473 = i16 16 ("A/D info.# A/D bits")
                  # "Pull out time stamp"
                  # "Save FIle"
                  n111 = case shown="0" w453 {
                    tunnel: w457 -> [w491 w493]
                    tunnel: [w490 w493] -> w456
                    tunnel: [w489 w492] -> w455
                    tunnel: w454 -> [w488 w492]
                    frame 0 {
                      n112 = Set File Position(refnum=w491, error in=w488) -> (refnum out=w490:refnum<file>, error out=w489:errorcluster)  [unwired: 2 in]
                    }
                    frame 1, Default {
                    }
                  }
                  n113 = Unbundle By Name(w487) -> ("rfpts"=w462:dbl, "rflines"=w459:dbl, "RcvBuffer"=w485:dbl)
                  n114 = Get File Position(4:w455, 7:w456) -> (0:w475:errorcluster, 2:w468:i64, 3:w476:refnum<file>)
                  n115 = expression code="x*2"(w459) -> (w458:dbl)
                  n116 = Compound Arithmetic op=MULTIPLY(w462, w459) -> (w469:dbl)
                  n117 = Add(x=w458, y=w468) -> (x+y=w464:dbl)
                  n118 = expression code="x*2"(w469) -> (w467:dbl)
                  n119 = Read from Binary File(5:w473, 8:w475, 10:w474, 11:w476) -> (0:w471:errorcluster, 2:w463:i16[], 3:w472:refnum<file>)  [unwired: 2 in, 1 out]
                  n120 = Set File Position(offset (in bytes) (0)=w464, refnum=w472, from (0:start)=w470, error in=w471) -> (refnum out=w466:refnum<file>, error out=w465:errorcluster)
                  n121 = Read from Binary File(5:w473, 8:w465, 10:w474, 11:w466) -> (0:w481:errorcluster, 2:w477:i16[], 3:w482:refnum<file>)  [unwired: 2 in, 1 out]
                  n122 = Add(x=w467, y=w468) -> (x+y=w478:dbl)
                  n123 = Build Array(w463, w477) -> (w460:i16[][])
                  n124 = Equal?(x=3, y=w485) -> (x = y?=w483:bool)
                  n125 = Set File Position(offset (in bytes) (0)=w478, refnum=w482, from (0:start)=w470, error in=w481) -> (refnum out=w480:refnum<file>, error out=w479:errorcluster)
                  n126 = Transpose 2D Array(2D array=w460) -> (transposed array=w461:i16[][])
                  n127 = call "VerasonicsTimeStamp.vi"("Array"=w461) -> ("Numeric"=w486:u32)  [unwired: 10 in]
                }
                frame "Save IQSumReal" {
                  # "Using scale values now in case GPU output is modified. Be careful of RF pts. Default IQ pt value is 1/2 of RF pts in final image.  Right now it is assumed that the Real output from GPU is sampled equal to sampling rate."
                  # "Real"
                  # "Pull out RcvData"
                  n128 = Unbundle By Name(w518) -> ("rfpts"=w502:dbl, "rflines"=w505:dbl, "RcvBuffer"=w499:dbl)
                  n129 = Set File Position(refnum=w513, from (0:start)=enum16{"start", "end", "current"}."current", error in=w512) -> (refnum out=w509:refnum<file>, error out=w510:errorcluster)  [unwired: 1 in]
                  n130 = Compound Arithmetic op=MULTIPLY(w502, w505) -> (w511:dbl)
                  n131 = Unbundle By Name(w495) -> ("IQFrame"=w494:dbl)
                  n132 = Read from Binary File(5:32 ("A/D info.# A/D bits"), 8:w510, 10:w511, 11:w509) -> (0:w503:errorcluster, 2:w519:i32[], 3:w504:refnum<file>)  [unwired: 2 in, 1 out]
                  n133 = Concatenate Strings("_SumReal" ("file name"), w506, w515) -> (w514:string)
                  n134 = Select(t=3, s=w497, f=w499) -> (s? t:f=w498:dbl)
                  n135 = Bundle By Name(cluster=w501, "A/D info.# bytes per A/D"=u16 4, "A/D info.# A/D bits"=u16 32 ("A/D info.TGC Flag")) -> (w523:T3)
                  n136 = call "NumberFileName.vi"("Digits"=w508, "File number"=w494, "file name"=w514) -> ("Numbered File"=w529:string)  [unwired: 1 in]
                  n137 = Concatenate Strings(w527, w529) -> (w528:string)
                  n138 = Build Path(base path=w526, name or relative path=w528) -> (appended path=w525:path)
                  n139 = call "MakeHeader.vi"("Header In"=w523) -> ("Header String"=w524:string)  [unwired: 6 in]
                  n140 = case shown="3" w498 {
                    tunnel: w525 -> [_ w537]
                    tunnel: w524 -> [_ w536]
                    tunnel: w519 -> [_ w535]
                    tunnel: [w530 w534] -> w517
                    tunnel: w503 -> [w530 w531]
                    frame 0, Default {
                    }
                    frame 3 {
                      w538 = FALSE ("prepend array or string size? (T)")
                      # "Save FIle"
                      n141 = Open/Create/Replace File(file path (use dialog)=w537, error in=w531, operation (0:open)=T5."replace or create") -> (refnum out=w541:refnum<file>, error out=w540:errorcluster)  [unwired: 3 in, 1 out]
                      n142 = Write to Binary File(file (use dialog)=w541, data=w536, error in=w540, 5:w538) -> (refnum out=w543:refnum<file>, error out=w542:errorcluster)  [unwired: 2 in, 1 out]
                      n143 = Write to Binary File(file (use dialog)=w543, data=w535, error in=w542, 5:w538) -> (refnum out=w533:refnum<file>, error out=w532:errorcluster)  [unwired: 2 in, 1 out]
                      n144 = Close File(refnum=w533, error in=w532) -> (error out=w534:errorcluster)  [unwired: 1 out]
                    }
                  }
                }
                frame "Save IQSum" {
                  # "Using scale values now in case GPU output is modified."
                  # "Real"
                  # "Save FIle"
                  # "Pull out RcvData"
                  n145 = case shown="Default" w562 {
                    tunnel: w561 -> [w590 w593]
                    tunnel: [w588 w592] -> w566
                    tunnel: w559 -> [w589 w591]
                    tunnel: [w587 w591] -> w558
                    frame "Verasonics" {
                      n146 = Unbundle By Name(w590) -> ("IQ_pts"=w588:dbl)
                      n147 = Bundle By Name(cluster=w589, "A/D info.# rf points per line"=w588) -> (w587:T3)
                    }
                    frame Default {
                      n148 = Unbundle By Name(w593) -> ("rfpts"=w592:dbl)
                    }
                  }
                  n149 = Unbundle By Name(w561) -> ("rflines"=w560:dbl, "RcvBuffer"=w555:dbl)
                  n150 = Select(t=u16 5 ("A/D info.# bytes per A/D"), s=w546, f=u16 9 ("A/D info.# bytes per A/D")) -> (s? t:f=w550:u16)
                  n151 = Compound Arithmetic op=MULTIPLY(w566, w560) -> (w570:dbl)
                  n152 = case shown="True" w565 {
                    tunnel: [w595 w631] -> w582
                    tunnel: [w605 w627] -> w578
                    tunnel: [w604 w626] -> w549
                    tunnel: [w603 w625] -> w577
                    tunnel: w573 -> [_ w624]
                    tunnel: w572 -> [w602 w623]
                    tunnel: w571 -> [w601 w622]
                    tunnel: w570 -> [w597 w609]
                    tunnel: w564 -> [w594 _]
                    tunnel: [w596 _] -> w563
                    frame True {
                      w606 = 32 ("A/D info.# A/D bits")
                      w598 = enum16{"start", "end", "current"}."current" ("from (0:start)")
                      n153 = Set File Position(refnum=w602, from (0:start)=w598, error in=w601) -> (refnum out=w599:refnum<file>, error out=w600:errorcluster)  [unwired: 1 in]
                      n154 = Read from Binary File(5:w606, 8:w600, 10:w597, 11:w599) -> (2:w605:i32[], 3:w595:refnum<file>)  [unwired: 2 in, 2 out]
                      n155 = Set File Position(refnum=w594, from (0:start)=w598) -> (refnum out=w607:refnum<file>, error out=w608:errorcluster)  [unwired: 2 in]
                      n156 = Read from Binary File(5:w606, 8:w608, 10:w597, 11:w607) -> (0:w603:errorcluster, 2:w604:i32[], 3:w596:refnum<file>)  [unwired: 2 in, 1 out]
                    }
                    frame False {
                      w628 = 32 ("A/D info.# A/D bits")
                      w611 = enum16{"start", "end", "current"}."start" ("from (0:start)")
                      n157 = Divide(x=w624, y=i64 2) -> (x/y=w621:dbl)
                      n158 = feedback #1() -> (w612:i64)
                      n159 = Add(x=w621, y=w612) -> (x+y=w619:dbl)
                      n160 = Set File Position(offset (in bytes) (0)=w612, refnum=w623, from (0:start)=w611, error in=w622) -> (refnum out=w613:refnum<file>, error out=w614:errorcluster)
                      n161 = Read from Binary File(5:w628, 8:w614, 10:w609, 11:w613) -> (0:w618:errorcluster, 2:w627:i32[], 3:w615:refnum<file>)  [unwired: 2 in, 1 out]
                      n162 = Get File Position(4:w618, 7:w615) -> (0:w617:errorcluster, 2:w620:i64, 3:w616:refnum<file>)
                      n163 = feedback-in #1(w620) -> ()
                      n164 = Set File Position(offset (in bytes) (0)=w619, refnum=w616, from (0:start)=w611, error in=w617) -> (refnum out=w629:refnum<file>, error out=w630:errorcluster)
                      n165 = Read from Binary File(5:w628, 8:w630, 10:w609, 11:w629) -> (0:w625:errorcluster, 2:w626:i32[], 3:w631:refnum<file>)  [unwired: 2 in, 1 out]
                    }
                  }
                  n166 = Unbundle By Name(w545) -> ("IQFrame"=w544:dbl)
                  n167 = Bundle By Name(cluster=w558, "A/D info.# bytes per A/D"=w550, "A/D info.# A/D bits"=u16 32 ("A/D info.TGC Flag")) -> (w579:T3)
                  n168 = Concatenate Strings("_IQSum" ("file name"), w567, w575) -> (w574:string)
                  n169 = Select(t=3, s=w556, f=w555) -> (s? t:f=w554:dbl)
                  n170 = call "NumberFileName.vi"("Digits"=w569, "File number"=w544, "file name"=w574) -> ("Numbered File"=w586:string)  [unwired: 1 in]
                  n171 = Concatenate Strings(w584, w586) -> (w585:string)
                  n172 = Select(t=i32[] [], s=w546, f=w549) -> (s? t:f=w547:i32[])
                  n173 = Build Path(base path=w583, name or relative path=w585) -> (appended path=w581:path)
                  n174 = call "MakeHeader.vi"("Header In"=w579) -> ("Header String"=w580:string)  [unwired: 6 in]
                  n175 = case shown="3" w554 {
                    tunnel: w581 -> [_ w640]
                    tunnel: w580 -> [_ w639]
                    tunnel: w578 -> [_ w636]
                    tunnel: w547 -> [_ w633]
                    tunnel: w577 -> [w632 w635]
                    tunnel: [w632 w634] -> w576
                    frame 0, Default {
                    }
                    frame 3 {
                      w641 = FALSE ("prepend array or string size? (T)")
                      # "Imaginary"
                      n176 = Open/Create/Replace File(file path (use dialog)=w640, error in=w635, operation (0:open)=T5."replace or create") -> (refnum out=w646:refnum<file>, error out=w645:errorcluster)  [unwired: 3 in, 1 out]
                      n177 = Write to Binary File(file (use dialog)=w646, data=w639, error in=w645, 5:w641) -> (refnum out=w648:refnum<file>, error out=w647:errorcluster)  [unwired: 2 in, 1 out]
                      n178 = Write to Binary File(file (use dialog)=w648, data=w636, error in=w647, 5:w641) -> (refnum out=w643:refnum<file>, error out=w642:errorcluster)  [unwired: 2 in, 1 out]
                      n179 = Write to Binary File(file (use dialog)=w643, data=w633, error in=w642, 5:w641) -> (refnum out=w638:refnum<file>, error out=w637:errorcluster)  [unwired: 2 in, 1 out]
                      n180 = Close File(refnum=w638, error in=w637) -> (error out=w634:errorcluster)  [unwired: 1 out]
                    }
                  }
                }
                frame "Save IQAll" {
                  # "Using scale values now in case GPU output is modified."
                  # "Real"
                  # "Save FIle"
                  # "Pull out RcvData"
                  n181 = case shown="Default" w667 {
                    tunnel: w666 -> [w695 w698]
                    tunnel: [w693 w697] -> w671
                    tunnel: w664 -> [w694 w696]
                    tunnel: [w692 w696] -> w663
                    frame "Verasonics" {
                      n182 = Unbundle By Name(w695) -> ("IQ_pts"=w693:dbl)
                      n183 = Bundle By Name(cluster=w694, "A/D info.# rf points per line"=w693) -> (w692:T3)
                    }
                    frame Default {
                      n184 = Unbundle By Name(w698) -> ("rfpts"=w697:dbl)
                    }
                  }
                  n185 = Unbundle By Name(w666) -> ("rflines"=w665:dbl, "RcvBuffer"=w660:dbl)
                  n186 = Select(t=u16 4 ("A/D info.# bytes per A/D"), s=w652, f=u16 9 ("A/D info.# bytes per A/D")) -> (s? t:f=w651:u16)
                  n187 = Compound Arithmetic op=MULTIPLY(w671, w665) -> (w675:dbl)
                  n188 = case shown="True" w670 {
                    tunnel: [w700 w736] -> w687
                    tunnel: [w710 w732] -> w682
                    tunnel: [w709 w731] -> w655
                    tunnel: [w708 w730] -> w681
                    tunnel: w677 -> [_ w729]
                    tunnel: w658 -> [w707 w716]
                    tunnel: w676 -> [w706 w728]
                    tunnel: w675 -> [w702 w717]
                    tunnel: w669 -> [w699 _]
                    tunnel: [w701 _] -> w668
                    frame True {
                      w711 = 32 ("A/D info.# A/D bits")
                      w703 = enum16{"start", "end", "current"}."current" ("from (0:start)")
                      n189 = Set File Position(refnum=w707, from (0:start)=w703, error in=w706) -> (refnum out=w704:refnum<file>, error out=w705:errorcluster)  [unwired: 1 in]
                      n190 = Read from Binary File(5:w711, 8:w705, 10:w702, 11:w704) -> (2:w710:i32[], 3:w700:refnum<file>)  [unwired: 2 in, 2 out]
                      n191 = Set File Position(refnum=w699, from (0:start)=w703) -> (refnum out=w712:refnum<file>, error out=w713:errorcluster)  [unwired: 2 in]
                      n192 = Read from Binary File(5:w711, 8:w713, 10:w702, 11:w712) -> (0:w708:errorcluster, 2:w709:i32[], 3:w701:refnum<file>)  [unwired: 2 in, 1 out]
                    }
                    frame False {
                      w733 = 32 ("A/D info.# A/D bits")
                      w719 = enum16{"start", "end", "current"}."start" ("from (0:start)")
                      n193 = Divide(x=w729, y=i64 2) -> (x/y=w727:dbl)
                      n194 = feedback #2() -> (w714:i64)
                      n195 = Add(x=w727, y=w714) -> (x+y=w726:dbl)
                      n196 = Set File Position(offset (in bytes) (0)=w714, refnum=w716, from (0:start)=w719, error in=w728) -> (refnum out=w720:refnum<file>, error out=w721:errorcluster)
                      n197 = Read from Binary File(5:w733, 8:w721, 10:w717, 11:w720) -> (0:w725:errorcluster, 2:w732:i32[], 3:w722:refnum<file>)  [unwired: 2 in, 1 out]
                      n198 = Get File Position(4:w725, 7:w722) -> (0:w724:errorcluster, 2:w715:i64, 3:w723:refnum<file>)
                      n199 = feedback-in #2(w715) -> ()
                      n200 = Set File Position(offset (in bytes) (0)=w726, refnum=w723, from (0:start)=w719, error in=w724) -> (refnum out=w734:refnum<file>, error out=w735:errorcluster)
                      n201 = Read from Binary File(5:w733, 8:w735, 10:w717, 11:w734) -> (0:w730:errorcluster, 2:w731:i32[], 3:w736:refnum<file>)  [unwired: 2 in, 1 out]
                    }
                  }
                  n202 = Bundle By Name(cluster=w663, "A/D info.# bytes per A/D"=w651, "A/D info.# A/D bits"=u16 32 ("A/D info.TGC Flag")) -> (w684:T3)
                  n203 = Concatenate Strings("_IQAll" ("file name"), w672, w679) -> (w678:string)
                  n204 = Unbundle By Name(w650) -> ("IQFrame"=w649:dbl)
                  n205 = Select(t=3, s=w661, f=w660) -> (s? t:f=w662:dbl)
                  n206 = call "NumberFileName.vi"("Digits"=w674, "File number"=w649, "file name"=w678) -> ("Numbered File"=w691:string)  [unwired: 1 in]
                  n207 = Concatenate Strings(w689, w691) -> (w690:string)
                  n208 = Select(t=i32[] [], s=w652, f=w655) -> (s? t:f=w657:i32[])
                  n209 = Build Path(base path=w688, name or relative path=w690) -> (appended path=w686:path)
                  n210 = call "MakeHeader.vi"("Header In"=w684) -> ("Header String"=w685:string)  [unwired: 6 in]
                  n211 = case shown="3" w662 {
                    tunnel: w686 -> [_ w745]
                    tunnel: w685 -> [_ w744]
                    tunnel: w682 -> [_ w741]
                    tunnel: w657 -> [_ w740]
                    tunnel: w681 -> [w737 w739]
                    tunnel: [w737 w738] -> w680
                    frame 0, Default {
                    }
                    frame 3 {
                      w746 = FALSE ("prepend array or string size? (T)")
                      # "Imaginary"
                      n212 = Open/Create/Replace File(file path (use dialog)=w745, error in=w739, operation (0:open)=T5."replace or create") -> (refnum out=w751:refnum<file>, error out=w750:errorcluster)  [unwired: 3 in, 1 out]
                      n213 = Write to Binary File(file (use dialog)=w751, data=w744, error in=w750, 5:w746) -> (refnum out=w753:refnum<file>, error out=w752:errorcluster)  [unwired: 2 in, 1 out]
                      n214 = Write to Binary File(file (use dialog)=w753, data=w741, error in=w752, 5:w746) -> (refnum out=w748:refnum<file>, error out=w747:errorcluster)  [unwired: 2 in, 1 out]
                      n215 = Write to Binary File(file (use dialog)=w748, data=w740, error in=w747, 5:w746) -> (refnum out=w743:refnum<file>, error out=w742:errorcluster)  [unwired: 2 in, 1 out]
                      n216 = Close File(refnum=w743, error in=w742) -> (error out=w738:errorcluster)  [unwired: 1 out]
                    }
                  }
                }
                frame "unused" {
                  w782 = 2.0  # double
                  w785 = 32 ("A/D info.# A/D bits")
                  # "Imaginary"
                  # "Real"
                  # "Save FIle"
                  # "Pull out RcvData"
                  n217 = Unbundle By Name(w779) -> ("IQ_pts"=w783:dbl, "rflines"=w793:dbl, "RcvBuffer"=w756:dbl)
                  n218 = Divide(x=w772, y=i64 2) -> (x/y=w767:dbl)
                  n219 = feedback #3() -> (w758:i64)  [unwired: 1 in]
                  n220 = Add(x=w767, y=w758) -> (x+y=w765:dbl)
                  n221 = Set File Position(offset (in bytes) (0)=w758, refnum=w770, from (0:start)=enum16{"start", "end", "current"}."start", error in=w769) -> (refnum out=w759:refnum<file>, error out=w760:errorcluster)
                  n222 = Multiply(x=w782, y=w783) -> (x*y=w784:dbl)
                  n223 = Multiply(x=w783, y=w793) -> (x*y=w768:dbl)
                  n224 = Read from Binary File(5:w785, 8:w760, 10:w768, 11:w759) -> (0:w764:errorcluster, 2:w781:i32[], 3:w761:refnum<file>)  [unwired: 2 in, 1 out]
                  n225 = Bundle By Name(cluster=w792, "A/D info.# rf points per line"=w784, "A/D info.# bytes per A/D"=u16 9, "A/D info.# A/D bits"=u16 32 ("A/D info.TGC Flag")) -> (w791:T3)
                  n226 = Concatenate Strings("_IQAll" ("file name"), w774) -> (w773:string)
                  n227 = Unbundle By Name(w755) -> ("IQFrame"=w754:dbl)
                  n228 = Get File Position(4:w764, 7:w761) -> (0:w763:errorcluster, 2:w766:i64, 3:w762:refnum<file>)
                  n229 = feedback-in #3(w766) -> ()
                  n230 = Set File Position(offset (in bytes) (0)=w765, refnum=w762, from (0:start)=enum16{"start", "end", "current"}."start", error in=w763) -> (refnum out=w788:refnum<file>, error out=w789:errorcluster)
                  n231 = call "NumberFileName.vi"("Digits"=w757, "File number"=w754, "file name"=w773) -> ("Numbered File"=w800:string)  [unwired: 1 in]
                  n232 = Read from Binary File(5:w785, 8:w789, 10:w768, 11:w788) -> (0:w778:errorcluster, 2:w780:i32[], 3:w796:refnum<file>)  [unwired: 2 in, 1 out]
                  n233 = Concatenate Strings(w798, w800) -> (w799:string)
                  n234 = Build Path(base path=w797, name or relative path=w799) -> (appended path=w795:path)
                  n235 = call "MakeHeader.vi"("Header In"=w791) -> ("Header String"=w794:string)  [unwired: 6 in]
                  n236 = case shown="3" w756 {
                    tunnel: w795 -> [_ w809]
                    tunnel: w794 -> [_ w808]
                    tunnel: w781 -> [_ w805]
                    tunnel: w780 -> [_ w804]
                    tunnel: w778 -> [w801 w803]
                    tunnel: [w801 w802] -> w777
                    frame 0, Default {
                    }
                    frame 3 {
                      w810 = FALSE ("prepend array or string size? (T)")
                      n237 = Open/Create/Replace File(file path (use dialog)=w809, error in=w803, operation (0:open)=T5."replace or create") -> (refnum out=w815:refnum<file>, error out=w814:errorcluster)  [unwired: 3 in, 1 out]
                      n238 = Write to Binary File(file (use dialog)=w815, data=w808, error in=w814, 5:w810) -> (refnum out=w817:refnum<file>, error out=w816:errorcluster)  [unwired: 2 in, 1 out]
                      n239 = Write to Binary File(file (use dialog)=w817, data=w805, error in=w816, 5:w810) -> (refnum out=w812:refnum<file>, error out=w811:errorcluster)  [unwired: 2 in, 1 out]
                      n240 = Write to Binary File(file (use dialog)=w812, data=w804, error in=w811, 5:w810) -> (refnum out=w807:refnum<file>, error out=w806:errorcluster)  [unwired: 2 in, 1 out]
                      n241 = Close File(refnum=w807, error in=w806) -> (error out=w802:errorcluster)  [unwired: 1 out]
                    }
                  }
                }
                frame "Save Img" {
                  n242 = Unbundle By Name(w823) -> ("IQPage"=w822:dbl)
                  n243 = Unbundle By Name(w819) -> ("IQFrame"=w818:dbl)
                  n244 = case shown="1" w822 {
                    tunnel: w823 -> [_ w858]
                    tunnel: w830 -> [_ w839]
                    tunnel: w829 -> [_ w853]
                    tunnel: w828 -> [w832 w851]
                    tunnel: w827 -> [w831 w850]
                    tunnel: [w832 w849] -> w826
                    tunnel: [w831 w846] -> w825
                    tunnel: w824 -> [_ w845]
                    tunnel: w821 -> [_ w837]
                    tunnel: w820 -> [_ w835]
                    tunnel: w818 -> [_ w833]
                    frame 0, Default {
                    }
                    frame 1 {
                      # "Only save page 1 cases. This is nod to Doppler"
                      # "Save FIle"
                      # "Pull out RcvData"
                      n245 = Unbundle By Name(w858) -> ("IQ_pts"=w844:dbl, "rflines"=w857:dbl, "RcvBuffer"=w834:dbl)
                      n246 = Concatenate Strings("_IMG" ("file name"), w837) -> (w836:string)
                      n247 = Set File Position(refnum=w851, from (0:start)=enum16{"start", "end", "current"}."current", error in=w850) -> (refnum out=w859:refnum<file>, error out=w860:errorcluster)  [unwired: 1 in]
                      n248 = Bundle By Name(cluster=w845, "A/D info.# rf points per line"=w844, "A/D info.# bytes per A/D"=u16 4, "A/D info.# A/D bits"=i16 32) -> (w843:T3)
                      n249 = Multiply(x=w844, y=w857) -> (x*y=w862:dbl)
                      n250 = call "NumberFileName.vi"("Digits"=w835, "File number"=w833, "file name"=w836) -> ("Numbered File"=w856:string)  [unwired: 1 in]
                      n251 = Read from Binary File(5:32 ("A/D info.# A/D bits"), 8:w860, 10:w862, 11:w859) -> (0:w847:errorcluster, 2:w840:i32[], 3:w849:refnum<file>)  [unwired: 2 in, 1 out]
                      n252 = Concatenate Strings(w839, w856) -> (w855:string)
                      n253 = Build Path(base path=w853, name or relative path=w855) -> (appended path=w854:path)
                      n254 = call "MakeHeader.vi"("Header In"=w843) -> ("Header String"=w852:string)  [unwired: 6 in]
                      n255 = case shown="1" w834 {
                        tunnel: FALSE ("prepend array or string size? (T)") -> [_ w875]
                        tunnel: w854 -> [_ w871]
                        tunnel: w852 -> [_ w870]
                        tunnel: w847 -> [w864 w867]
                        tunnel: [w864 w866] -> w846
                        tunnel: w840 -> [_ w865]
                        frame 0, Default {
                        }
                        frame 1 {
                          n256 = Open/Create/Replace File(file path (use dialog)=w871, error in=w867, operation (0:open)=T5."replace or create") -> (refnum out=w874:refnum<file>, error out=w873:errorcluster)  [unwired: 3 in, 1 out]
                          n257 = Write to Binary File(file (use dialog)=w874, data=w870, error in=w873, 5:w875) -> (refnum out=w877:refnum<file>, error out=w876:errorcluster)  [unwired: 2 in, 1 out]
                          n258 = Write to Binary File(file (use dialog)=w877, data=w865, error in=w876, 5:w875) -> (refnum out=w869:refnum<file>, error out=w868:errorcluster)  [unwired: 2 in, 1 out]
                          n259 = Close File(refnum=w869, error in=w868) -> (error out=w866:errorcluster)  [unwired: 1 out]
                        }
                      }
                    }
                  }
                }
              }
            }
          }
        }
        frame True {
        }
      }
    }
    n260 = Index Array(array=w45) -> (element=w46:u32)  [unwired: 1 in]
    n261 = case shown="\"Save RF\", Default" "Enum" {
      tunnel: w65 -> [_ w101]
      tunnel: w64 -> [_ w100]
      tunnel: "Split files?" -> [_ w99]
      tunnel: w48 -> [_ w98]
      frame "None" {
      }
      frame "Save RF", Default {
        n262 = case shown="True" w99 {
          tunnel: w98 -> [_ w102]
          frame False {
          }
          frame True {
            n263 = Close File(refnum=w102) -> ()  [unwired: 1 in, 2 out]
          }
        }
        n264 = Close File(refnum=w100, error in=w101) -> ()  [unwired: 2 out]
      }
    }
    n265 = Subtract(x=w45, y=w46) -> (x-y=w43:u32[])
    n266 = Divide(x=w43, y=sgl 40.0) -> (x/y=w42:sgl[])
    "time stamp" <- w42
  }
  n267 = Array Size(array=w10) -> (size(s)=w9:i32)
  n268 = Decrement(x=w9) -> (x-1=w8:i32)
  n269 = for {
    N: w8 -> [_]
    tunnel: w10 -> [w886] mode=indexing
    tunnel: w10 -> [w888]
    tunnel: [w885] -> w11 mode=indexing
    i -> [w884]
    n270 = Increment(x=w884) -> (x+1=w889:i32)
    n271 = Index Array(array=w888, index=w889) -> (element=w887:sgl)
    n272 = Subtract(x=w887, y=w886) -> (x-y=w885:sgl)
  }
  "time diff" <- w11
